vi "run script line.vi"(8 "error in (no error)":errorcluster caption="에러 입력(에러 없음)", 11 "Script Line 입력":refnum<class "Script Line.lvclass">) -> (0 "error out":errorcluster caption="에러 출력", 2 "log":string, 3 "Script Line 출력":refnum<class "Script Line.lvclass">)   [LabVIEW 2020, in "Script Line.lvclass"]
uses:
  Script Line.lvclass
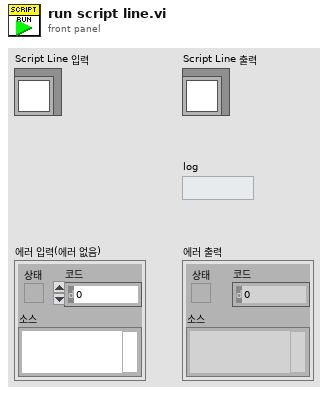
[diagram p1: front panel]
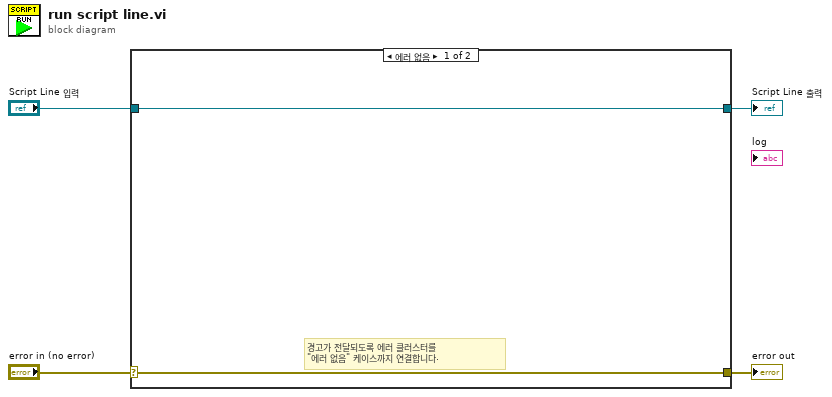
[diagram p0: block diagram]
diagram:
  n1 = case shown="에러 없음" "error in (no error)" {
    selector: "error in (no error)" -> [w5 w8]
    tunnel: [w5 w8] -> w3
    tunnel: [w6 w7] -> w1
    tunnel: "Script Line 입력" -> [w6 w7]
    frame No Error {
      # "경고가 전달되도록 에러 클러스터를\n\"에러 없음\" 케이스까지 연결합니다."
    }
    frame Error {
    }
  }
  "error out" <- w3
  "Script Line 출력" <- w1
